vi "ABF_Read.vi"(4 "error in (no error)":errorcluster, 7 "Path of ABF file":path=path "D:/bme/abffile/demo3.abf") -> (0 "error out":errorcluster, 2 "File Paramters":T2, 3 "Whole Trace":sgl[][](graph))   [LabVIEW 2017]
panel:
  out "channel number":i32
  out "Header":T1
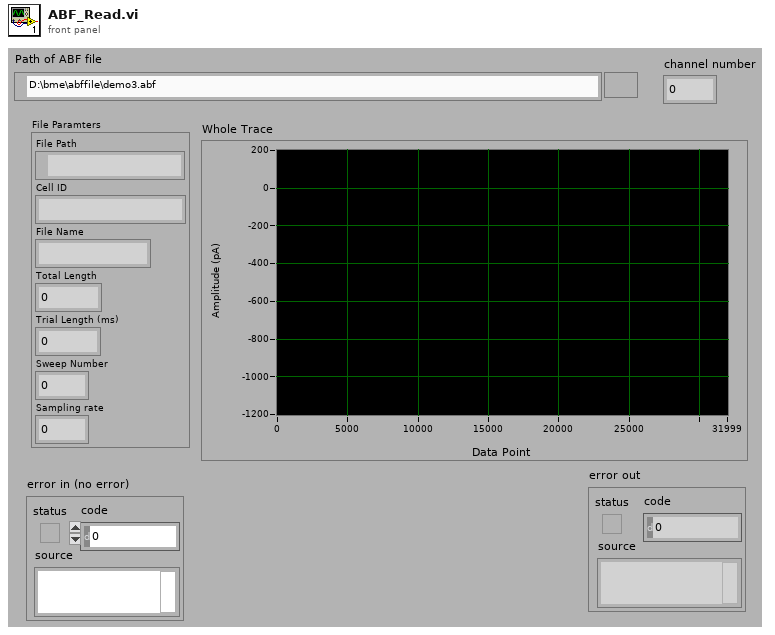
[diagram p1: front panel]
types:
  T1 = cluster{"AbfFormat":string, "fFileVersionNumber":sgl, "nOperationMode":i8, "IActualAcqLength":u32, "fNumPointsIgnored":i8, "IActualEpisodes":i32, "fADCSampleInterval":sgl, "INumSamplesPerEpisode":u32, "IEpisodesPerRun":u32, "fADCRange":sgl, "IADCResolution":u32}
  T2 = cluster{"File Path":path, "Cell ID":string, "File Name":string, "Total Length":i32, "Trial Length (ms)":dbl, "Sweep Number":dbl, "Sampling rate":dbl}
  T3 = enum16{"big-endian, network order", "native, host order", "little-endian"}
  T4 = cluster{"NumSamplePerEpisode":u32, "sweepCount":u32, "dataRate":i32}
  T5 = cluster{"stripped path":path, "name":string, "name":string, u32, "NumSamplePerEpisode":u32, "sweepCount":u32, "dataRate":i32}
  T6 = cluster{"stripped path":path, "name":string, "name":string, dbl, dbl, dbl, "sampling rate":dbl}
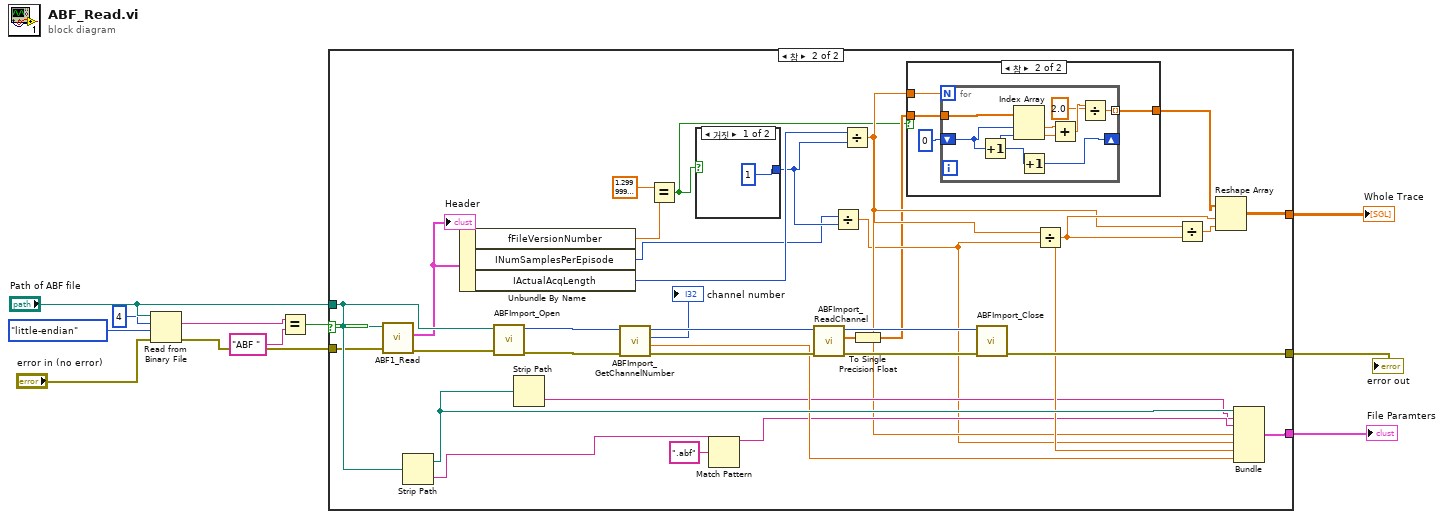
[diagram p0: block diagram]
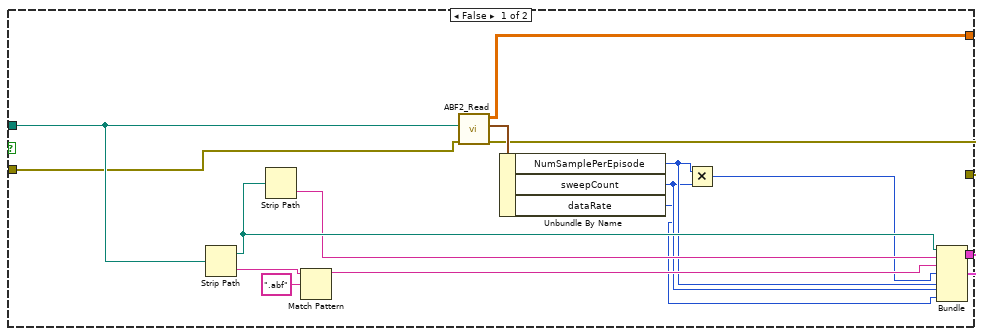
[diagram p2: hidden frame]
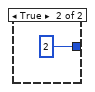
[diagram p4: hidden frame]
diagram:
  n1 = Read from Binary File(8:"error in (no error)", 9:T3."little-endian" ("바이트 순서(0:big-endian, network order)"), 10:4 ("카운트(1)"), 11:"Path of ABF file") -> (0:w6:errorcluster, 2:w3:string)  [unwired: 2 in, 2 out]
  n2 = Equal?(x=w3, y="ABF ") -> (x = y?=w2:bool)
  n3 = case shown="참" w2 {
    tunnel: [w19 w54] -> w1
    tunnel: "Path of ABF file" -> [w25 w42]
    tunnel: [w23 w50] -> w11
    tunnel: w6 -> [w13 w41]
    tunnel: [w12 w48] -> w10
    frame False {
      n4 = Strip Path(path=w25) -> (stripped path=w22:path, name=w24:string)
      n5 = Strip Path(path=w22) -> (name=w21:string)  [unwired: 1 out]
      n6 = Match Pattern(string=w24, regular expression=".abf" ("정규식")) -> (before substring=w20:string)  [unwired: 1 in, 3 out]
      n7 = call "ABF2_Read.vi"("에러 입력"=w13, "FilePath"=w25) -> ("error out"=w12:errorcluster, "DataProperties"=w18:T4, "DataArray"=w19:sgl[][])  [unwired: 3 in]
      n8 = Unbundle By Name(w18) -> ("NumSamplePerEpisode"=w16:u32, "sweepCount"=w15:u32, "dataRate"=w14:i32)
      n9 = Multiply(x=w16, y=w15) -> (x*y=w17:u32)
      n10 = Bundle("stripped path"=w22, "name"=w21, "name"=w20, w17, "NumSamplePerEpisode"=w16, "sweepCount"=w15, "dataRate"=w14) -> (w23:T5)  [unwired: 1 in]
    }
    frame True {
      n11 = call "ABF1_Read.vi"("에러 입력"=w41, "FilePath"=w42) -> ("error out"=w40:errorcluster, "Header"=w39:T1)  [unwired: 4 in]
      "Header" <- w39
      n12 = Strip Path(path=w42) -> (stripped path=w51:path, name=w49:string)
      n13 = Unbundle By Name(w39) -> ("fFileVersionNumber"=w31:sgl, "INumSamplesPerEpisode"=w33:u32, "IActualAcqLength"=w36:u32)
      n14 = call "ABFImport_Open.vi"("error in (no error)"=w40, "abf file path"=w42) -> ("error out"=w57:errorcluster, "reference number"=w58:i32)  [unwired: 8 in]
      n15 = Strip Path(path=w51) -> (name=w44:string)  [unwired: 1 out]
      n16 = call "ABFImport_GetChannelNumber.vi"("error in (no error)"=w57, "reference number"=w58) -> ("error out"=w55:errorcluster, "sampling rate"=w47:dbl, "channel number"=→"channel number":i32, "reference out"=w56:i32)  [unwired: 6 in]
      n17 = Equal?(x=sgl 1.3, y=w31) -> (x = y?=w27:bool)
      n18 = case shown="거짓" w27 {
        tunnel: [u32 1 ("y") u32 2 ("y")] -> w34
        frame False {
        }
        frame True {
        }
      }
      n19 = Match Pattern(string=w49, regular expression=".abf" ("정규식")) -> (before substring=w45:string)  [unwired: 1 in, 3 out]
      n20 = call "ABFImport_ReadChannel.vi"("error in (no error)"=w55, "reference number"=w56) -> ("error out"=w59:errorcluster, "signal"=w37:sgl[], "reference out"=w52:i32)  [unwired: 7 in]
      n21 = Divide(x=w33, y=w34) -> (x/y=w32:dbl)
      n22 = Divide(x=w36, y=w34) -> (x/y=w35:dbl)
      n23 = To Single Precision Float(number=w37) -> (single precision float=w29:sgl[])
      n24 = case shown="참" w27 {
        tunnel: w35 -> [_ w63]
        tunnel: w29 -> [w60 w62]
        tunnel: [w60 w61] -> w28
        frame False {
        }
        frame True {
          n25 = for {
            N: w63 -> [_]
            tunnel: w62 -> [w73]
            shift-right: [w70] -> _
            shift-left: u32 0 ("y") -> [w72]
            tunnel: [w65] -> w61 mode=indexing
            n26 = Increment(x=w72) -> (x+1=w71:u32)
            n27 = Index Array(array=w73, index #1=w72, index #2=w71) -> (element #1=w69:sgl, element #2=w68:sgl)
            n28 = Increment(x=w71) -> (x+1=w70:u32)
            n29 = Add(x=w69, y=w68) -> (x+y=w67:sgl)
            n30 = Divide(x=w67, y=sgl 2.0) -> (x/y=w65:sgl)
          }
        }
      }
      n31 = call "ABFImport_Close.vi"("error in (no error)"=w59, "reference number"=w52) -> ("error out"=w48:errorcluster)  [unwired: 9 in]
      n32 = Divide(x=w35, y=w32) -> (x/y=w46:dbl)
      n33 = Divide(x=w35, y=w46) -> (x/y=w53:dbl)
      n34 = Reshape Array(w28, w46, w53) -> (w54:sgl[][])
      n35 = Bundle("stripped path"=w51, "name"=w44, "name"=w45, w35, w32, w46, "sampling rate"=w47) -> (w50:T6)  [unwired: 1 in]
    }
  }
  "Whole Trace" <- w1
  "File Paramters" <- w11
  "error out" <- w10
